vi "pullTxTimestamps.vi"(8 "error in (no error)":errorcluster, 11 "Modbus in":refnum<class "Modbus.lvclass">) -> (0 "error out":errorcluster, 2 "Timestamp":u64[](array[numeric]), 3 "Modbus out":refnum<class "Modbus.lvclass">)   [LabVIEW 2016, in "RTModbusFPGA.lvlib" / "Modbus.lvclass"]
uses:
  Modbus.lvclass
  Modbus.lvclass/Modbus.ctl
  Common_RT_FPGA/IReadU64FIFO/IReadU64FIFO.lvclass
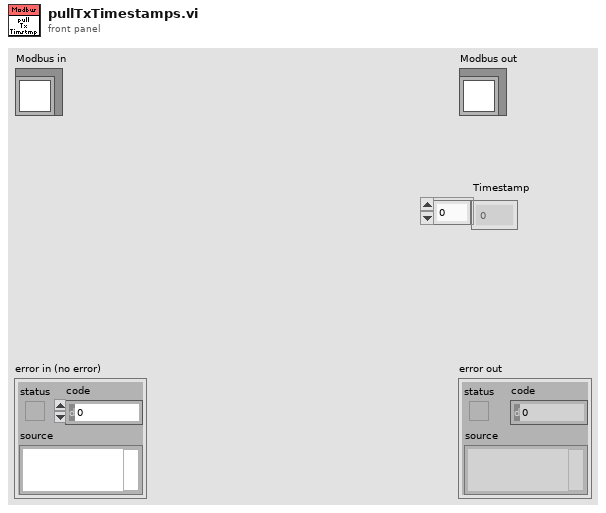
[diagram p1: front panel]
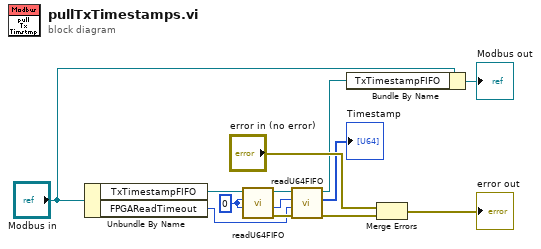
[diagram p0: block diagram]
diagram:
  w11 = u32 0 ("NumberOfElements")
  n1 = Unbundle By Name("Modbus in") -> ("TxTimestampFIFO"=w3:refnum<class "IReadU64FIFO.lvclass">, "FPGAReadTimeout"=w7:i32)
  n2 = call-dynamic "readU64FIFO.vi"("Timeout"=w11, "NumberOfElements"=w11, "IReadU64FIFO in"=w3) -> ("error out"=w10:errorcluster, "ElementsRemaining"=w8:u32, "IReadU64FIFO out"=w9:refnum<class "IReadU64FIFO.lvclass">)  [unwired: 5 in, 1 out]
  n3 = call-dynamic "readU64FIFO.vi"("error in (no error)"=w10, "Timeout"=w7, "NumberOfElements"=w8, "IReadU64FIFO in"=w9) -> ("error out"=w6:errorcluster, "Data"=→"Timestamp":u64[], "IReadU64FIFO out"=w2:refnum<class "IReadU64FIFO.lvclass">)  [unwired: 4 in, 1 out]
  n4 = Bundle By Name(cluster="Modbus in", "TxTimestampFIFO"=w2) -> (→"Modbus out":refnum<class "Modbus.lvclass">)
  n5 = Merge Errors("error in (no error)", w6) -> (→"error out":errorcluster)
